vi "Read Dinero.vi"(8 "error in (no error)":errorcluster, 11 "Dinero in":refnum<class "Dinero.lvclass">) -> (0 "error out":errorcluster, 2 "Dinero":refnum<vi>, 3 "Dinero out":refnum<class "Dinero.lvclass">)   [LabVIEW 2020, in "Dinero.lvlib" / "Dinero.lvclass"]
uses:
  Dinero.lvclass
  Dinero.lvclass/Dinero.ctl
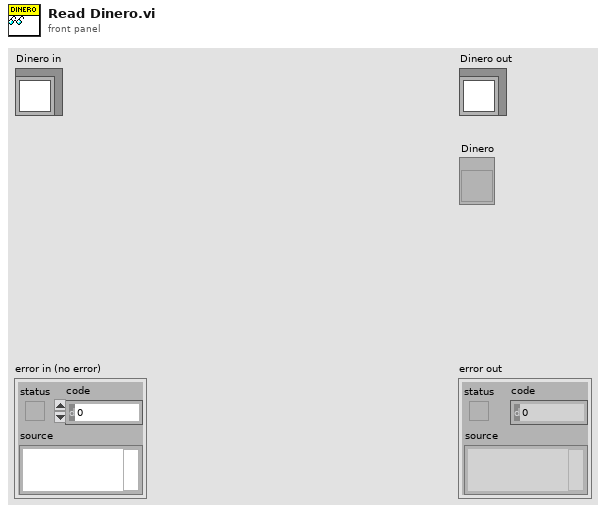
[diagram p1: front panel]
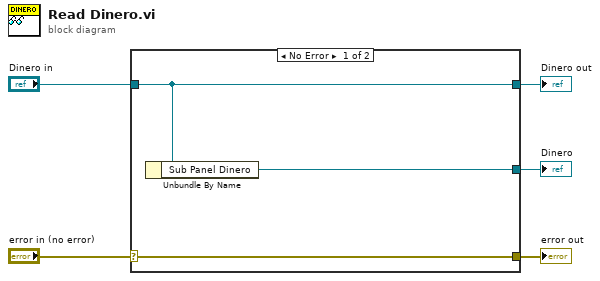
[diagram p0: block diagram]
diagram:
  n1 = case shown="No Error" "error in (no error)" {
    selector: "error in (no error)" -> [w8 w9]
    tunnel: [w8 w9] -> w4
    tunnel: [w7 w10] -> w2
    tunnel: "Dinero in" -> [w7 w10]
    tunnel: [w6 _] -> w1
    frame No Error {
      n2 = Unbundle By Name(w7) -> ("Sub Panel Dinero"=w6:refnum<vi>)
    }
    frame Error {
    }
  }
  "error out" <- w4
  "Dinero out" <- w2
  "Dinero" <- w1
